vi "VCS Set Motor Parameter.vi"(8 "error in (no error)":errorcluster, 10 "motor Data":T1={"motor Type"=1, "continuousCurrent"=1000, "peakCurrent"=1000, "polePair"=1, "thermalTimeConstant"=40} {"motor Type" items=["Phase modulated DC motor "=1, "Sinusoidal PM BL motor"=10, "Trapezoidal PM BL motor"=11]}, 11 "axis in":cluster{"keyHandle":u32, "nodeId":u16}={"keyHandle"=0, "nodeId"=1}) -> (0 "error out":errorcluster, 3 "axis out":cluster{"keyHandle":u32, "nodeId":u16}={"keyHandle"=0, "nodeId"=1})   [LabVIEW 2010]
doc: "<B>VCS Set Motor Parameter</B> writes all motor parameters."
uses:
  Resources/EposCmd.dll
  Resources/EposCmd64.dll
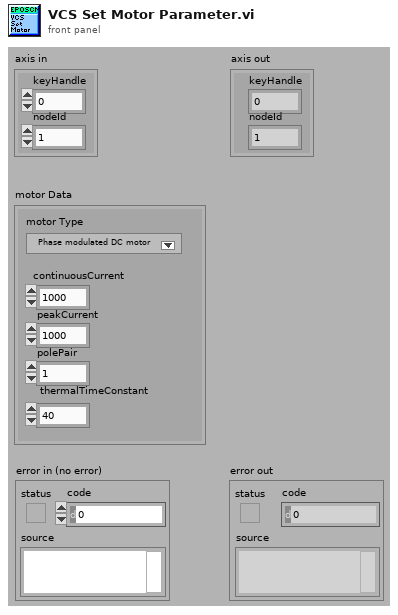
[diagram p1: front panel]
types:
  T1 = cluster{"motor Type":u16, "continuousCurrent":u16, "peakCurrent":u16, "polePair":u8, "thermalTimeConstant":u16}
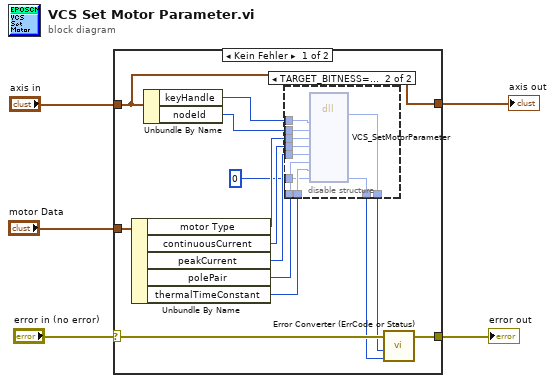
[diagram p0: block diagram]
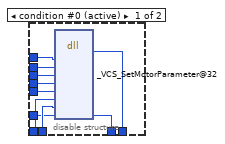
[diagram p2: hidden frame]
diagram:
  n1 = case shown="Kein Fehler" "error in (no error)" {
    selector: "error in (no error)" -> [w19 w41]
    tunnel: [w18 w41] -> w4
    tunnel: "motor Data" -> [w16 _]
    tunnel: "axis in" -> [w8 w40]
    tunnel: [w8 w40] -> w1
    frame No Error {
      n2 = Unbundle By Name(w16) -> ("motor Type"=w15:u16, "continuousCurrent"=w14:u16, "peakCurrent"=w13:u16, "polePair"=w12:u8, "thermalTimeConstant"=w11:u16)
      n3 = Unbundle By Name(w8) -> ("keyHandle"=w10:u32, "nodeId"=w9:u16)
      n4 = disable-structure shown="TARGET_BITNESS==64" {
        disable-tunnel: [w29 w39] -> w17
        disable-tunnel: w15 -> [w28 w38]
        disable-tunnel: w14 -> [w27 w37]
        disable-tunnel: w13 -> [w26 w36]
        disable-tunnel: w12 -> [w25 w35]
        disable-tunnel: w11 -> [w24 w34]
        disable-tunnel: w10 -> [w23 w33]
        disable-tunnel: w9 -> [w22 w32]
        disable-tunnel: u32 0 ("pErrorCode") -> [w21 w31]
        disable-tunnel: [w20 w30] -> w6
        frame condition #0 (active) {
          n5 = dll-call lib="C:/Sources/LabView/maxon EPOS/Resources/EposCmd.*" fn="_VCS_SetMotorParameter@32"("KeyHandle"=w23, "NodeId"=w22, "MotorType"=w28, "ContinuousCurrent"=w27, "PeakCurrent"=w26, "PolePair"=w25, "ThermalTimeConstant"=w24, "pErrorCode"=w21) -> (w20:i32, "pErrorCode"=w29:u32)  [unwired: 10 in, 2 out]
        }
        frame condition #1 {
          n6 = dll-call lib="C:/setup/Resources/EposCmd64.*" fn="VCS_SetMotorParameter" ("EposCmd.dll:_VCS_SetMotorParameter@32")("KeyHandle"=w33, "NodeId"=w32, "MotorType"=w38, "ContinuousCurrent"=w37, "PeakCurrent"=w36, "PolePair"=w35, "ThermalTimeConstant"=w34, "pErrorCode"=w31) -> ("Rückgabetyp"=w30:i32, "pErrorCode"=w39:u32)  [unwired: 10 in, 2 out]
        }
      }
      n7 = call "Error Converter (ErrCode or Status).vi"("error code"=w17, "return type"=w6, "error in (no error)"=w19) -> ("error out"=w18:errorcluster)  [unwired: 7 in]
    }
    frame Error {
    }
  }
  "error out" <- w4
  "axis out" <- w1
